vi "Ej_3_Indicador_Tabla.vi"() -> ()   [LabVIEW 2021]
panel:
  in  "stop":bool
  out "Table Control":string[][](table)
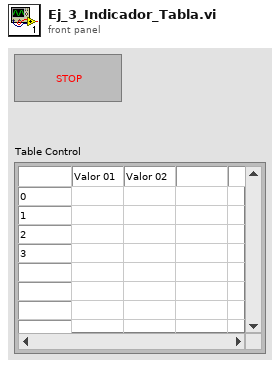
[diagram p1: front panel]
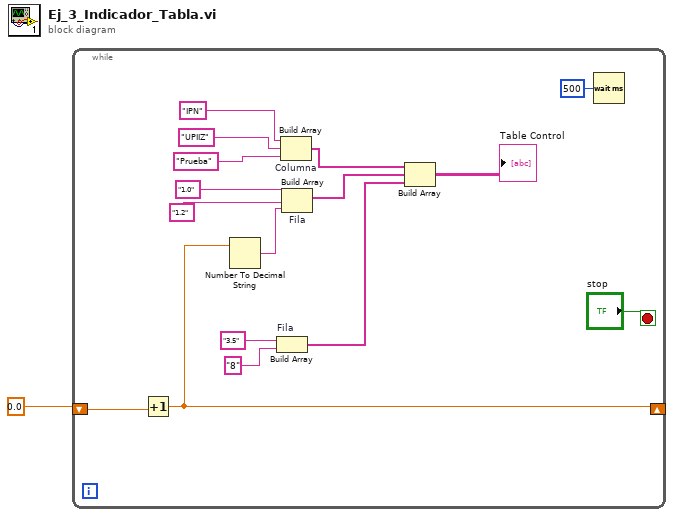
[diagram p0: block diagram]
diagram:
  n1 = while {
    shift-right: [w2] -> _
    shift-left: 0.0 -> [w3]
    stop <- "stop" stop-if-true
    n2 = Increment(x=w3) -> (x+1=w2:dbl)
    n3 = Number To Decimal String(number=w2) -> (decimal integer string=w4:string)  [unwired: 1 in]
    n4 = Build Array "Fila"("3.5" ("element"), "8" ("element")) -> (w7:string[])
    n5 = Build Array "Columna"("IPN", "UPIIZ", "Prueba" ("element")) -> (w16:string[])
    n6 = Build Array "Fila"("1.0", "1.2", w4) -> (w15:string[])
    n7 = Build Array(w16, w15, w7) -> (→"Table Control":string[][])
    n8 = Wait (ms)(milliseconds to wait=u32 500) -> ()  [unwired: 1 out]
  }
